vi "Main_TestStand.vi"() -> ()   [LabVIEW 2019]
uses:
  <vilib>/ptbypt/NI_PtbyPt.lvlib
panel:
  out "motor 1 correction":dbl(graph)
  out "Labview PID Inputs (should not match gains) 2":T1
  in  "Proportional Gain (Kc) 2":dbl
  in  "Derivative Gain (Kd) 2":dbl format="%#_13g"
  in  "Integral Gain (Ki) 2":dbl format="%#_13g"
  in  "Integral Gain (Ki)":dbl format="%#_13g"
  in  "Derivative Gain (Kd)":dbl format="%#_13g"
  out "Labview PID Inputs (should not match gains)":T1
  in  "Proportional Gain (Kc)":dbl
  out "Raw x value":dbl(graph)
  in  "Adjustment x":dbl format="%0.2f"
  in  "Adjustment y":dbl format="%0.2f"
  out "Raw y value":i16(graph)
  in  "low cutoff freq y":dbl=0.01 format="%#_13g"
  in  "low cutoff freq x":dbl=0.01 format="%#_13g"
  out "Filtered Correction y":dbl format="%0.2f"
  out "Filtered Correction x":dbl format="%0.2f"
  out "Filtered Correction y":dbl(graph)
  out "Filtered Correction x":dbl(graph)
  out "Motor 2 Correction":dbl
  out "Motor 1 Correction":dbl
  out "error out":errorcluster
  out "error out 2":errorcluster
  out "error out 5":errorcluster
  out "error out 6":errorcluster
  in  "Initial Motor Power":dbl
  in  "Boolean":bool
  # "X-Axis Gains"
  # "Y-Axis Gains"
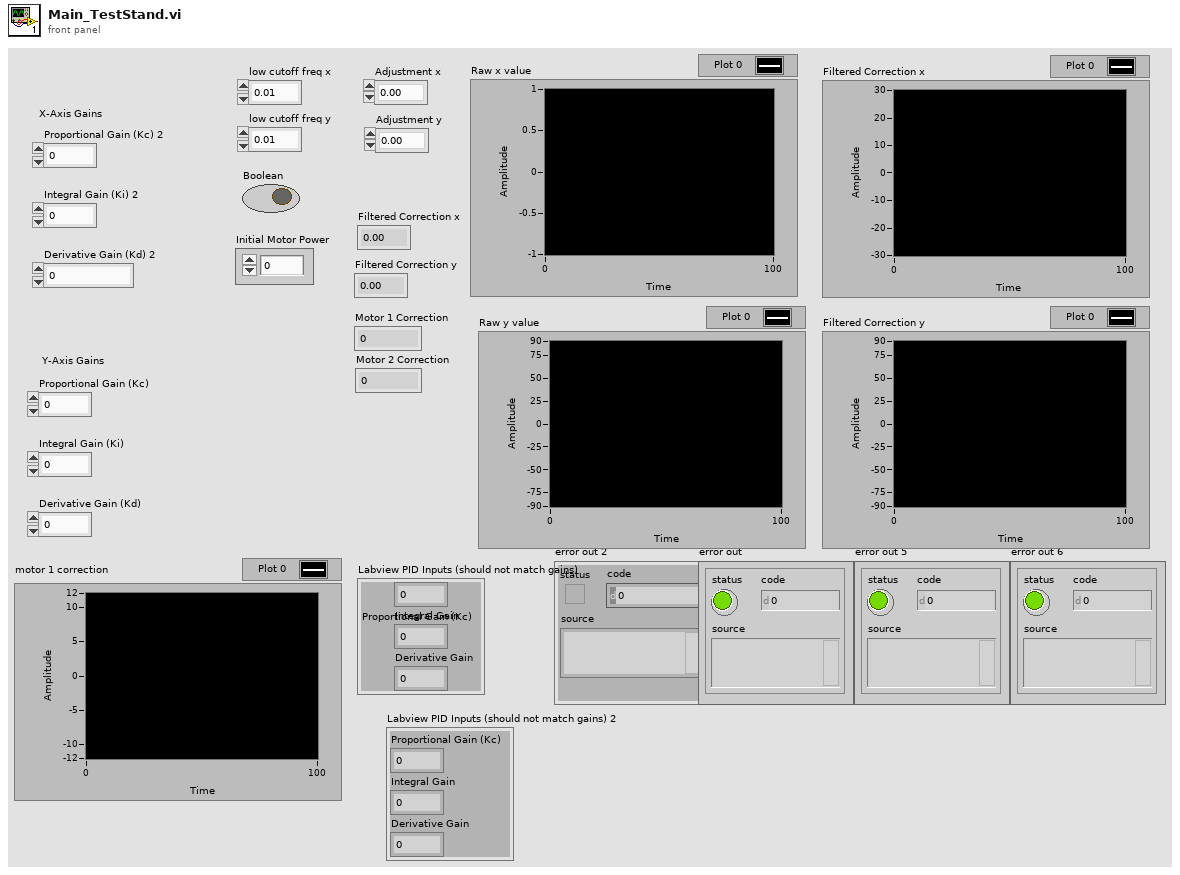
[diagram p1: front panel]
types:
  T1 = cluster{"Proportional Gain (Kc)":dbl, "Integral Gain":dbl, "Derivative Gain":dbl}
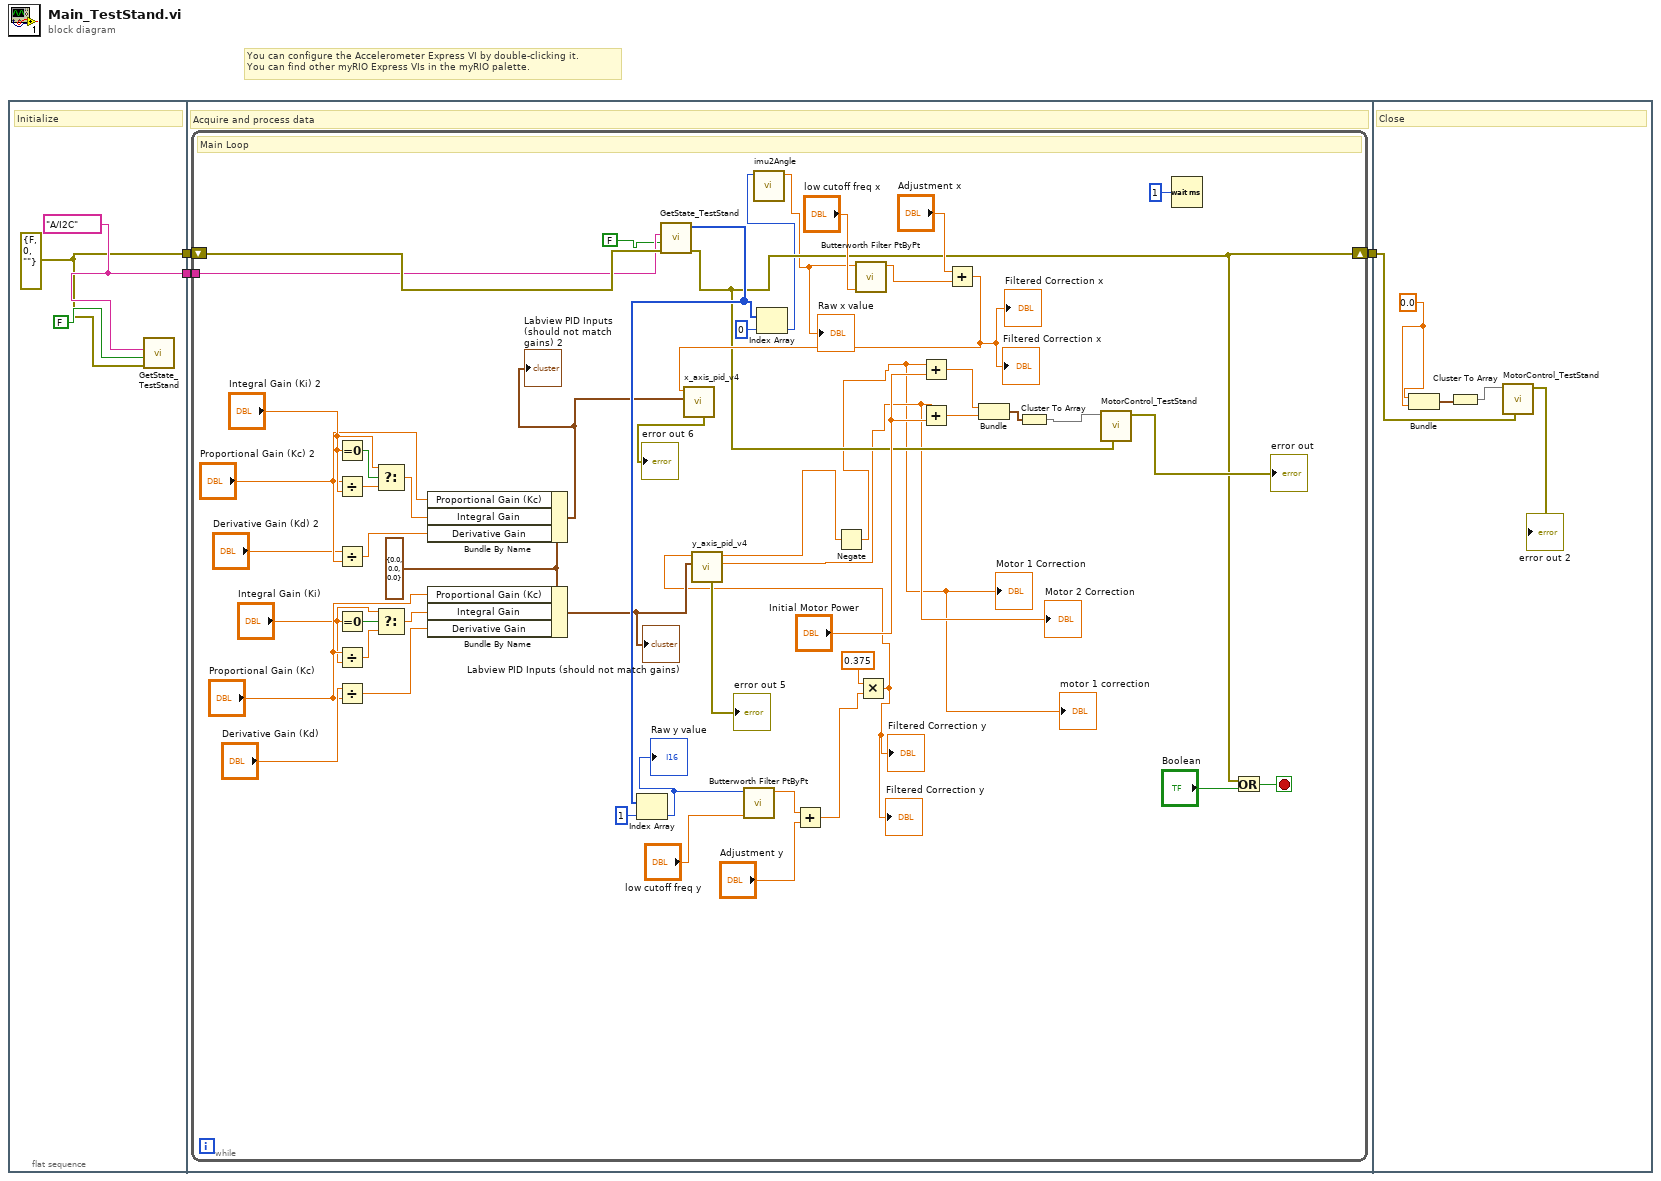
[diagram p0: block diagram]
diagram:
  # "You can configure the Accelerometer Express VI by double-clicking it.\nYou can find other myRIO Express VIs in the myRIO palette."
  n1 = flat-sequence {
    tunnel: [w6] -> w3
    tunnel: [w4] -> w2
    tunnel: [w9] -> w1
    tunnel: w3 -> [w8]
    tunnel: w2 -> [w7]
    tunnel: w1 -> [w62]
    frame #0 {
      w6 = tag "A/I2C" ("IMU Channel")
      w4 = errorcluster {"status"=FALSE, "code"=0, "source"=""} ("error in (no error)")
      # "Initialize"
      n2 = call "GetState_TestStand.vi"("error in (no error)"=w4, "Calibrate?"=FALSE, "IMU Channel"=w6) -> ()  [unwired: 4 in, 3 out]
    }
    frame #1 {
      # "Acquire and process data"
      n3 = while {
        shift-right: [w35] -> w9
        shift-left: w7 -> [w39]
        tunnel: w8 -> [w38]
        stop <- w60 stop-if-true
        w17 = T1 {"Proportional Gain (Kc)"=0.0, "Integral Gain"=0.0, "Derivative Gain"=0.0} ("PID Gains (x-axis)")
        # "Main Loop"
        n4 = Equal To 0?(x="Integral Gain (Ki) 2") -> (x = 0?=w21:bool)
        n5 = Divide(x="Proportional Gain (Kc) 2", y="Integral Gain (Ki) 2") -> (x/y=w23:dbl)
        n6 = Divide(x="Derivative Gain (Kd) 2", y="Proportional Gain (Kc) 2") -> (x/y=w19:dbl)
        n7 = Equal To 0?(x="Integral Gain (Ki)") -> (x = 0?=w28:bool)
        n8 = Divide(x="Proportional Gain (Kc)", y="Integral Gain (Ki)") -> (x/y=w26:dbl)
        n9 = Divide(x="Derivative Gain (Kd)", y="Proportional Gain (Kc)") -> (x/y=w30:dbl)
        n10 = Select(t="Integral Gain (Ki) 2", s=w21, f=w23) -> (s? t:f=w24:dbl)
        n11 = Select(t="Integral Gain (Ki)", s=w28, f=w26) -> (s? t:f=w25:dbl)
        n12 = Bundle By Name(cluster=w17, "Proportional Gain (Kc)"="Proportional Gain (Kc) 2", "Integral Gain"=w24, "Derivative Gain"=w19) -> (w16:T1)
        "Labview PID Inputs (should not match gains) 2" <- w16
        n13 = Bundle By Name(cluster=w17, "Proportional Gain (Kc)"="Proportional Gain (Kc)", "Integral Gain"=w25, "Derivative Gain"=w30) -> (w32:T1)
        "Labview PID Inputs (should not match gains)" <- w32
        n14 = call "GetState_TestStand.vi"("error in (no error)"=w39, "Calibrate?"=FALSE, "IMU Channel"=w38) -> ("error out"=w35:errorcluster, "imu accel"=w36:i16[])  [unwired: 4 in, 1 out]
        n15 = Index Array(array=w36, index=1) -> (element=w50:i16)
        "Raw y value" <- w50
        n16 = call <vilib>:"Butterworth Filter PtByPt.vi"("low cutoff freq: fl"="low cutoff freq y", "x"=w50) -> ("Filtered x"=w49:dbl)  [unwired: 7 in, 1 out]
        n17 = Index Array(array=w36, index=0) -> (element=w11:i16)
        n18 = call "imu2Angle.vi"("Sensor Input"=w11) -> ("Angle (radians)"=w10:dbl)  [unwired: 10 in]
        "Raw x value" <- w10
        n19 = Add(x=w49, y="Adjustment y") -> (x+y=w13:dbl)
        n20 = call <vilib>:"Butterworth Filter PtByPt.vi"("low cutoff freq: fl"="low cutoff freq x", "x"=w10) -> ("Filtered x"=w47:dbl)  [unwired: 7 in, 1 out]
        n21 = Multiply(x=0.375, y=w13) -> (x*y=w12:dbl)
        "Filtered Correction y" <- w12
        "Filtered Correction y" <- w12
        n22 = call "y_axis_pid_v4.vi"("PID Gains"=w32, "Y In"=w12) -> ("Motor 2"=w34:dbl, "Motor 1"=w33:dbl, "error out"=→"error out 5":errorcluster)  [unwired: 5 in, 2 out]
        "Motor 2 Correction" <- w34
        n23 = Negate(x=w33) -> (-x=w15:dbl)
        "Motor 1 Correction" <- w15
        "motor 1 correction" <- w15
        n24 = Add(x=w15, y="Initial Motor Power") -> (x+y=w54:dbl)
        n25 = Add(x=w34, y="Initial Motor Power") -> (x+y=w53:dbl)
        n26 = Add(x="Adjustment x", y=w47) -> (x+y=w43:dbl)
        "Filtered Correction x" <- w43
        "Filtered Correction x" <- w43
        n27 = call "x_axis_pid_v4.vi"("PID Gains"=w16, "X In"=w43) -> ("error out"=→"error out 6":errorcluster)  [unwired: 5 in, 4 out]
        n28 = Bundle(w54, w53) -> (w40:cluster{dbl, dbl})  [unwired: 1 in]
        n29 = Cluster To Array(cluster=w40) -> (array=w41:dbl[])
        n30 = call "MotorControl_TestStand.vi"("error in (no error)"=w35, "Array"=w41) -> ("error out"=→"error out":errorcluster)  [unwired: 9 in]
        n31 = Wait (ms)(milliseconds to wait=u32 1) -> ()  [unwired: 1 out]
        n32 = Or(x=w35, y="Boolean") -> (x .or. y?=w60:bool)
      }
    }
    frame #2 {
      w65 = 0.0
      # "Close"
      n33 = Bundle(w65, w65) -> (w64:cluster{dbl, dbl})  [unwired: 1 in]
      n34 = Cluster To Array(cluster=w64) -> (array=w63:dbl[])
      n35 = call "MotorControl_TestStand.vi"("error in (no error)"=w62, "Array"=w63) -> ("error out"=→"error out 2":errorcluster)  [unwired: 9 in]
    }
  }
